vi "dsdll_enumerate_devices_querry_list.vi"(8 "error in":errorcluster, 9 "device count":i32, 10 "device list object":u8[](array[numeric]), 11 "dsdll instance in":T1) -> (0 "error out":errorcluster, 2 "device list":T2[](array[typedef]), 3 "dsdll instance out":T1)   [LabVIEW 2018, in "dsdll.lvlib"]
doc: "Querys output or capture device records from device list."
uses:
  dsdll.lvlib
  dsdll_device_record.ctl
  dsdll_instance.ctl
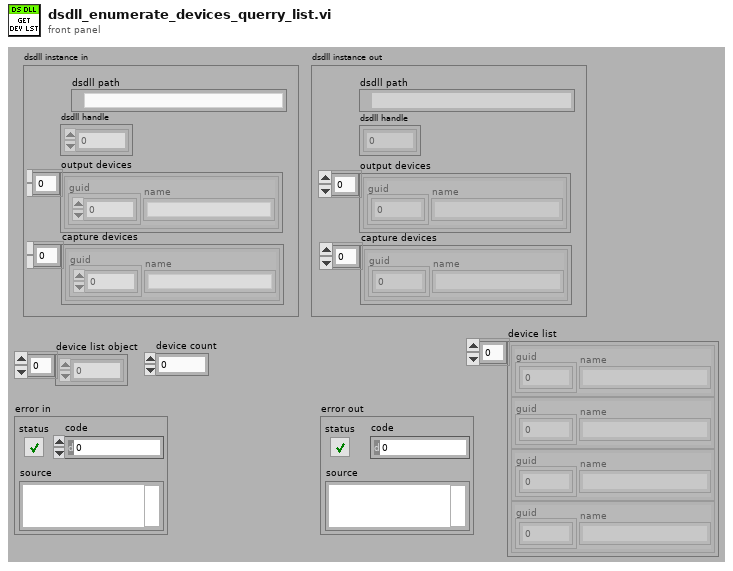
[diagram p1: front panel]
types:
  T1 = typedef "dsdll.lvlib/dsdll_instance.ctl" = cluster{"dsdll path":path, "dsdll handle":u8[], "output devices":T2[], "capture devices":T2[]}
  T2 = typedef "dsdll.lvlib/dsdll_device_record.ctl" = cluster{"guid":u8[], "name":string}
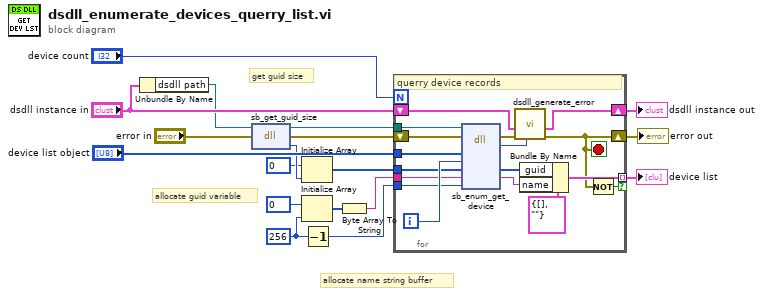
[diagram p0: block diagram]
diagram:
  w12 = 256 ("dimension size")
  # "allocate name string buffer"
  # "allocate guid variable"
  # "get guid size"
  n1 = Unbundle By Name("dsdll instance in") -> ("dsdll path"=w1:path)
  n2 = dll-call lib="dsdll.dll" fn="sb_get_guid_size" ("sb_get_handle_size()")(path in=w1, error in="error in") -> (path out=w5:path, error out=w4:errorcluster, "size [B]"=w7:u32)  [unwired: 1 in]
  n3 = Initialize Array(u8 0, w7) -> (w8:u8[])
  n4 = Initialize Array(u8 0, w12) -> (w10:u8[])
  n5 = Decrement(x=w12) -> (x-1=w13:i32)
  n6 = Byte Array To String(unsigned byte array=w10) -> (string=w11:string)
  n7 = for {
    N: "device count" -> [_]
    shift-right: [w19] -> w15
    shift-left: w4 -> [w35]
    shift-right: [w32] -> w16
    shift-left: "dsdll instance in" -> [w33]
    tunnel: w5 -> [w30]
    tunnel: w8 -> [w28]
    tunnel: w11 -> [w27]
    tunnel: w13 -> [w26]
    tunnel: "device list object" -> [w25]
    tunnel: [w21] -> w17 mode=indexing if=w20
    i -> [w29]
    stop <- w19 stop-if-true
    # "querry device records"
    n8 = dll-call lib="dsdll.dll" fn="sb_enum_get_device" ("sb_get_handle_size()")(path in=w30, error in=w35, "dev_list"=w25, "dev_id"=w29, "guid"=w28, "str"=w27, "strlen"=w26) -> (error out=w34:errorcluster, "error"=w31:i32, "guid"=w23:u8[], "str"=w22:string)  [unwired: 4 in, 1 out]
    n9 = call "dsdll_generate_error.vi"("error code"=w31, "error in"=w34, "dsdll instance in"=w33) -> ("error out"=w19:errorcluster, "dsdll instance out"=w32:T1)  [unwired: 6 in, 1 out]
    n10 = Bundle By Name(cluster=T2 {"guid"=[], "name"=""} ("DS device"), "guid"=w23, "name"=w22) -> (w21:T2)
    n11 = Not(x=w19) -> (.not. x?=w20:bool)
  }
  "device list" <- w17
  "dsdll instance out" <- w16
  "error out" <- w15
